vi "GetScrapped.vi"(8 "error in":errorcluster, 11 "ProductUnit in":refnum<class "ProductUnit.lvclass">) -> (0 "error out":errorcluster, 2 "Scrapped":bool, 3 "ProductUnit out":refnum<class "ProductUnit.lvclass">)   [LabVIEW 2021, in "ProligentXMLGenerator.lvlib" / "ProductUnit.lvclass"]
doc: "Flag representing whether the product unit has been scrapped or not. When not specified, it is assumed that the product unit is not scrapped."
uses:
  ProductUnit.lvclass
  ProductUnit.lvclass/ProductUnit.ctl
  Base/Attribute/Attribute.lvclass
  Base/Boolean/Boolean.lvclass
  C:/Projects/proligent-xml-generator-labview/src/ProligentXMLGenerator/Base/Attribute/Attribute.lvclass
  C:/Projects/proligent-xml-generator-labview/src/ProligentXMLGenerator/Base/Boolean/Boolean.lvclass
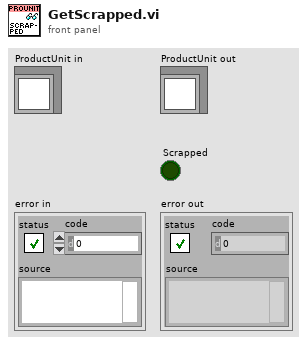
[diagram p1: front panel]
types:
  T1 = typedef "ProligentXMLGenerator.lvlib/ProductUnit.lvclass/Data.ctl" = cluster{"Name":string, "Characteristics":refnum<class "Characteristic.lvclass">[], "Documents":refnum<class "Document.lvclass">[], "CustomData":refnum<class "CustomData.lvclass">, "ProductUnitIdentifier":refnum<class "NonEmptyString_50.lvclass">, "ProductFullName":refnum<class "FullName.lvclass">, "Scrapped":refnum<class "Boolean.lvclass">, "ScrappedTime":refnum<class "DateTime.lvclass">, "CreationTime":refnum<class "DateTime.lvclass">, "ManufacturingTime":refnum<class "DateTime.lvclass">, "ByManufacturer":refnum<class "NonEmptyString_255.lvclass">, "TimeZoneInfoId":string}
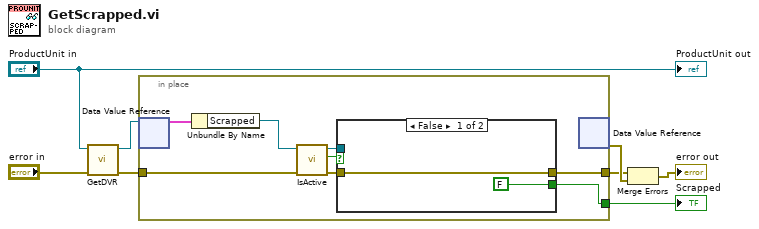
[diagram p0: block diagram]
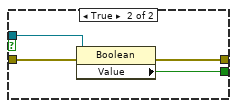
[diagram p2: hidden frame]
diagram:
  n1 = call "GetDVR.vi"("error in"="error in", "ProductUnit in"="ProductUnit in") -> ("error out"=w2:errorcluster, "DVRReference"=w7:refnum<data-value>)  [unwired: 8 in]
  n2 = in-place "In Place Element Structure" {
    in-place-border: [w15] -> w6
    in-place-border: w2 -> [w12]
    in-place-border: [w14] -> w1
    n3 = in-place-dvr #1(w7) -> (w16:T1)  [unwired: 1 out]
    n4 = Unbundle By Name(w16) -> ("Scrapped"=w11:refnum<class "Boolean.lvclass">)
    n5 = call "IsActive.vi"("error in"=w12, "Attribute in"=w11) -> ("error out"=w13:errorcluster, "IsActive"=w9:bool, "Attribute in"=w10:refnum<class "Boolean.lvclass">)  [unwired: 7 in]
    n6 = case shown="False" w9 {
      tunnel: [FALSE w22] -> w15
      tunnel: [w17 w21] -> w14
      tunnel: w13 -> [w17 w20]
      tunnel: w10 -> [_ w19]
      frame False {
      }
      frame True {
        n7 = property on="Property Node" class="Boolean"(reference=w19, error in=w20) -> (error out=w21:errorcluster, "Value"=w22:bool)  [unwired: 1 out]
      }
    }
    n8 = in-place-dvr #1() -> (w8:errorcluster)  [unwired: 1 in, 1 out]
  }
  "Scrapped" <- w6
  n9 = Merge Errors(w1, w8) -> (→"error out":errorcluster)
  "ProductUnit out" <- "ProductUnit in"
